vi "Periodic Tasks.vi"(8 "error in":errorcluster) -> ()   [LabVIEW 2017]
doc: "This VI runs in parallel to other tasks. It can contain as many user-defined periodic loops as you need. These can carry out PID or other sorts of timed response."
uses:
  <vilib>/Rock Robotics/WPI/Solenoid/WPI_SolenoidValue.ctl
  <vilib>/Rock Robotics/WPI/DriverStation/WPI_DriverStationRobotMode2.ctl
  <vilib>/Rock Robotics/WPI/ThirdParty/Phoenix-LabVIEW/Motor Controller/Controls/CTRE_Phoenix_MotorControl_ControlMode.ctl
  LabVIEW_is_Under_Control.lib/Util/Toggle/Change Detect.vi
  LabVIEW_is_Under_Control.lib/Util/Toggle/Change Detect Boolean.vi
  Robot Global Data.vi
  <vilib>/Rock Robotics/Network Tables/NT Write String.vi
  <vilib>/Rock Robotics/Network Tables/NT Write Number.vi
  <vilib>/Rock Robotics/WPI/Solenoid/WPI_SolenoidSetEnum.vi
  <vilib>/Rock Robotics/Network Tables/NT Write Boolean.vi
  <vilib>/Rock Robotics/Network Tables/NT Read Boolean.vi
panel:
  in  "Holding? Time":dbl=1000.0 format="%#_13g"
  out "Elevador Encoder":dbl
  out "Yaw":dbl
  in  "Exchange":dbl=4.0
  in  "ScoringHigh":dbl=80.0
  in  "Scoring Low":dbl=67.0
  in  "Enable squared":bool
  in  "Score":dbl=-0.3
  in  "Segurando":dbl=0.3
  in  "Expelir":dbl=-0.3
  in  "Coletar":dbl=0.9
  # "Para alterar:\n\nAlternar velocidade entre exchange e switch/scale\n\nNão deixar cancelar enquanto está cancelando"
  # "Intake"
  # "Drivetrain"
  # "Elevador"
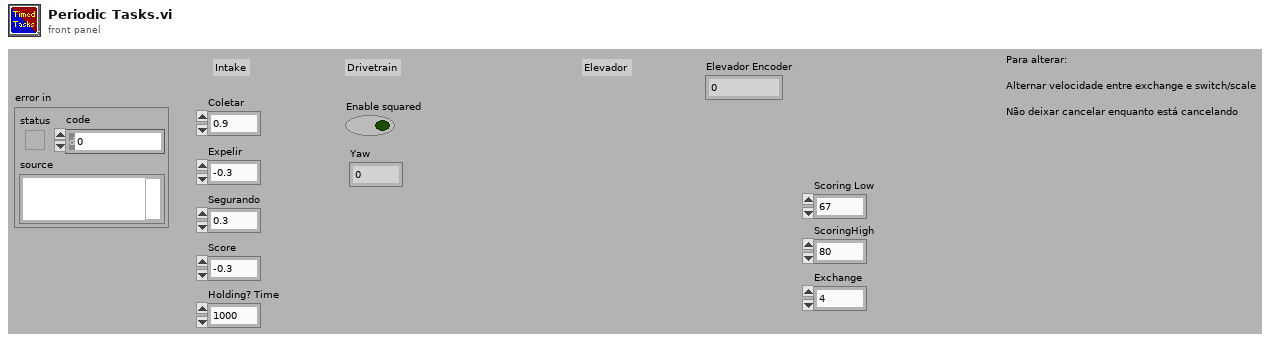
[diagram p1: front panel]
types:
  T1 = typedef "Máquina de estado do elevador.ctl" = enum16{"Resting", "Scoring Low", "Scoring Higher", "Exchange"}
  T2 = enum16{"Repouso", "Coletando", "Segurando", "Score"}
  T3 = typedef "WPI_EncoderDevRef.ctl" = cluster{"DevStatus":errorcluster, "EncoderIndex":T4, "CounterIndex":T5, "DistancePerCount":dbl, "Decoding Type":T6}
  T4 = typedef "FPGA_EncoderIdx.ctl" = enum8{"Enc 0", "Enc 1", "Enc 2", "Enc 3", "Enc 4", "Enc 5", "Enc 6", "Enc 7", "Invalid"}
  T5 = typedef "FPGA_CounterCtrSystemIndex.ctl" = enum8{"Ctr 0", "Ctr 1", "Ctr 2", "Ctr 3", "Ctr 4", "Ctr 5", "Ctr 6", "Ctr 7", "Invalid"}
  T6 = typedef "WPI_EncoderType.ctl" = enum16{"1x", "2x", "4x"}
  T7 = typedef "WPI_SwitchDevRef.ctl" = cluster{"DevStatus":errorcluster, "DIO Channel":T8, "CntIndex":T5, "Normally Closed":bool}
  T8 = typedef "FPGA_DIOChannel.ctl" = enum8{"DIO 0", "DIO 1", "DIO 2", "DIO 3", "DIO 4", "DIO 5", "DIO 6", "DIO 7", "DIO 8", "DIO 9", "DIO MXP 0", "DIO MXP 1", "DIO MXP 2", "DIO MXP 3", "DIO MXP 4", "DIO MXP 5", "DIO MXP 6", "DIO MXP 7", "DIO MXP 8", "DIO MXP 9", "DIO MXP 10", "DIO MXP 11", "DIO MXP 12", "DIO MXP 13", "DIO MXP 14", "DIO MXP 15", "SPI Port CS1", "SPI Port CS2", "SPI Port CS3", "SPI Port MISO", "SPI Port MOSI", "Invalid"}
  T9 = typedef "WPI_SolenoidDevRef.ctl" = cluster{"DevStatus":errorcluster, "Pneumatics Control Module":u8, "Forward Solenoid Channel":T10, "Reverse Solenoid Channel":T10}
  T10 = typedef "WPI_SolenoidChannel.ctl" = enum8{"Solenoid 0", "Solenoid 1", "Solenoid 2", "Solenoid 3", "Solenoid 4", "Solenoid 5", "Solenoid 6", "Solenoid 7", "Invalid"}
  T11 = typedef "WPI_MotorControlDeviceRef.ctl" = cluster{"DeviceStatus":errorcluster, "Type":T12, "PWM":cluster{"PWM Channel":T13, "DeadBand":T14}, "CAN":cluster{"Device Number":u8, "SetOutput VI Ref":variant, "GetOutput VI Ref":variant, "Enable VI Ref":variant, "Disable VI Ref":variant, "Data":variant}, "Invert":bool, "DIO PWM":cluster{"PWM \"Enable\" Channel":T13, "DIOChannel":T8, "PWM Rate":dbl}}
  T12 = typedef "WPI_MotorControlType.ctl" = enum16{"PWM", "CAN", "DIO PWM"}
  T13 = typedef "FPGA_DIOPWMChannel.ctl" = enum8{"PWM 0", "PWM 1", "PWM 2", "PWM 3", "PWM 4", "PWM 5", "PWM 6", "PWM 7", "PWM 8", "PWM 9", "PWM MXP 0", "PWM MXP 1", "PWM MXP 2", "PWM MXP 3", "PWM MXP 4", "PWM MXP 5", "PWM MXP 6", "PWM MXP 7", "PWM MXP 8", "PWM MXP 9", "Invalid"}
  T14 = typedef "WPI_PWMDeadband.ctl" = cluster{"Name":string, "maxPositivePwm":i32, "minPositivePwm":i32, "centerPwm":i32, "maxNegativePwm":i32, "minNegativePwm":i32, "angularRange":u16}
  T15 = cluster{"Yaw":dbl, "Roll":dbl, "Pitch":dbl, "Heading":dbl, "Fused Heading":dbl}
  T16 = typedef "WPI_SolenoidValue.ctl" = enum16{"Off", "On", "Forward", "Reverse"}
  T17 = typedef "WPI_DriverStationRobotMode2.ctl" = enum16{"Autonomous Disabled", "Autonomous Enabled", "Teleop Disabled", "Teleop Enabled", "Disconnected", "Finish", "Test Disabled", "Test Enabled", "Emergency Stopped"}
  T18 = typedef "Button Cluster.ctl" = cluster{"Buttons[0]":bool, "Buttons[1]":bool, "Buttons[2]":bool, "Buttons[3]":bool, "Buttons[4]":bool, "Buttons[5]":bool, "Buttons[6]":bool, "Buttons[7]":bool, "Buttons[8]":bool, "Buttons[9]":bool}
  T19 = typedef "CTRE_Phoenix_MotorControl_ControlMode.ctl" = u16
  T20 = typedef "Axes Cluster.ctl" = cluster{"Axes[0]":dbl, "Axes[1]":dbl, "Axes[2]":dbl, "Axes[3]":dbl, "Axes[4]":dbl, "Axes[5]":dbl, "Axes[6]":dbl, "Axes[7]":dbl, "Axes[8]":dbl}
  T21 = typedef "D-Pad.ctl" = cluster{"Top":bool, "Bottom":bool, "None":bool, "Right":bool, "Left":bool}
  T22 = cluster{"proportional gain (Kc)":dbl, "integral time (Ti, min)":dbl, "derivative time (Td, min)":dbl}
  T23 = enum16{"Coletar", "Expelir", "Chao", "Down", "Up", "Resting"}
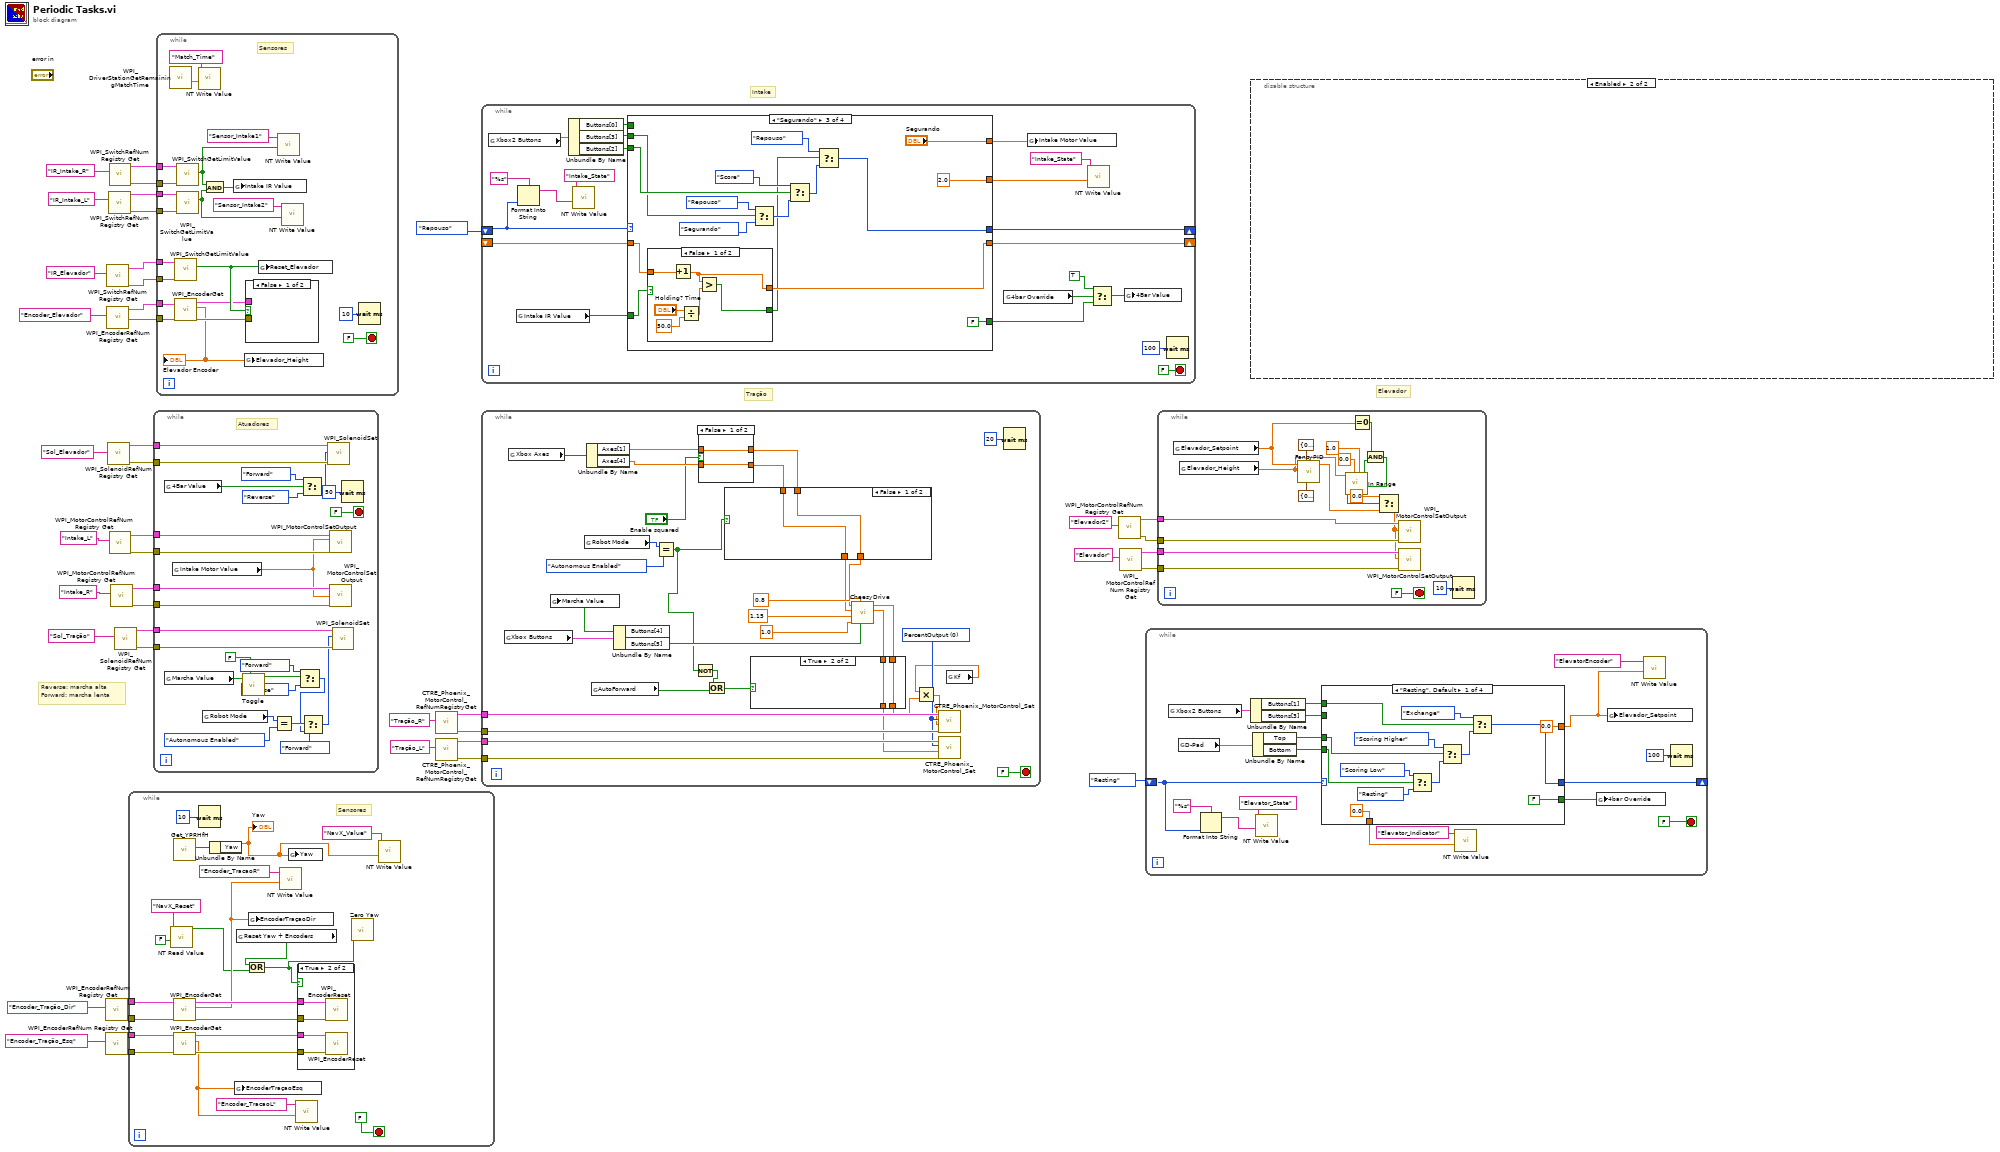
[diagram p0: block diagram]
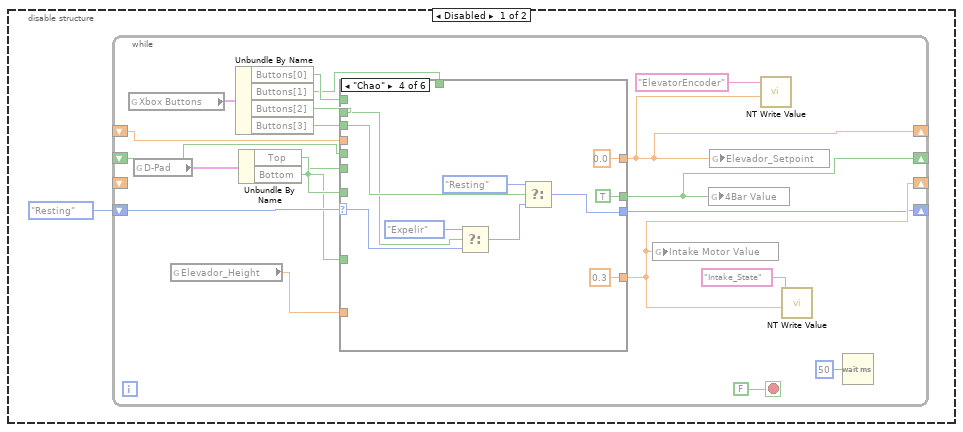
[diagram p2: hidden frame]
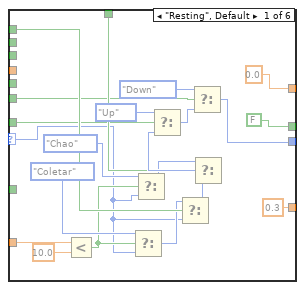
[diagram p3: hidden frame]
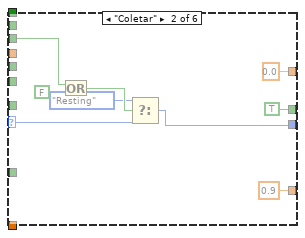
[diagram p4: hidden frame]
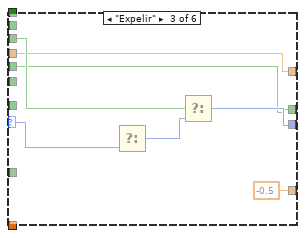
[diagram p5: hidden frame]
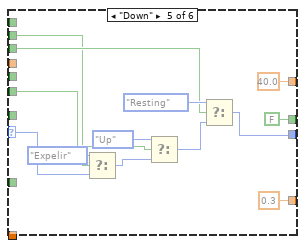
[diagram p6: hidden frame]
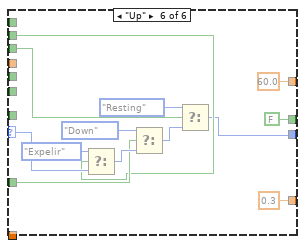
[diagram p7: hidden frame]
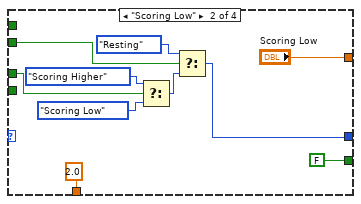
[diagram p9: hidden frame]
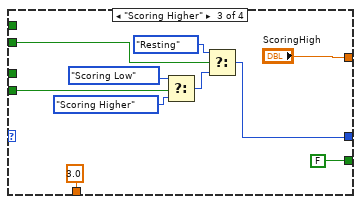
[diagram p10: hidden frame]
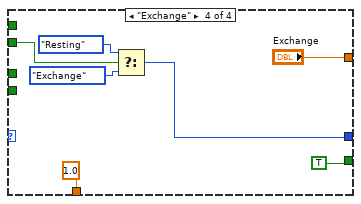
[diagram p11: hidden frame]
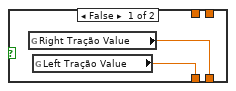
[diagram p12: hidden frame]
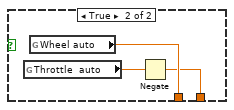
[diagram p13: hidden frame]
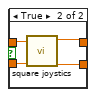
[diagram p14: hidden frame]
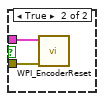
[diagram p15: hidden frame]
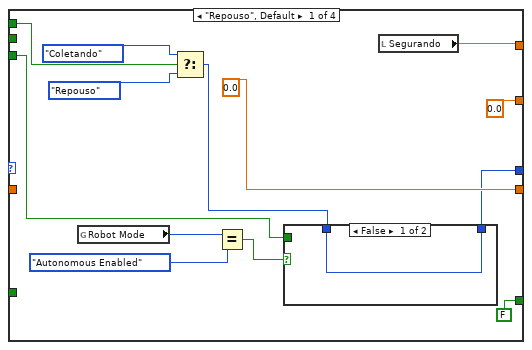
[diagram p16: hidden frame]
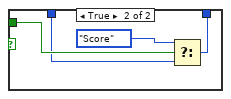
[diagram p17: hidden frame]
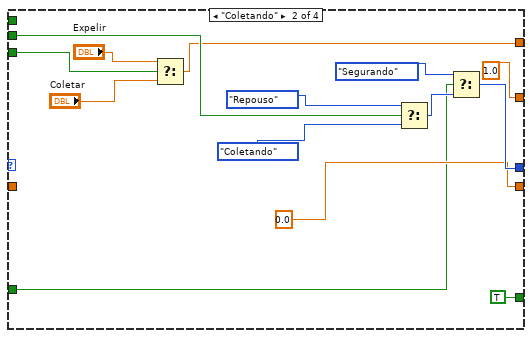
[diagram p18: hidden frame]
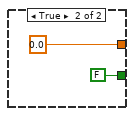
[diagram p19: hidden frame]
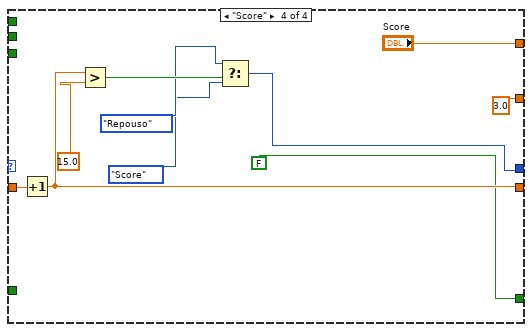
[diagram p20: hidden frame]
diagram:
  # "Reverse: marcha alta\nForward: marcha lenta"
  # "Elevador"
  # "Tração"
  # "Intake"
  n1 = call <vilib>:"WPI_EncoderRefNum Registry Get.vi"("refnum name"="Encoder_Tração_Dir") -> ("error out"=w8:errorcluster, "EncoderDevRef"=w9:T3)  [unwired: 9 in]
  n2 = call <vilib>:"WPI_EncoderRefNum Registry Get.vi"("refnum name"="Encoder_Tração_Esq") -> ("error out"=w7:errorcluster, "EncoderDevRef"=w6:T3)  [unwired: 9 in]
  n3 = call <vilib>:"WPI_SwitchRefNum Registry Get.vi"("refnum name"="IR_Elevador") -> ("error out"=w19:errorcluster, "SwitchDevRef"=w20:T7)  [unwired: 9 in]
  n4 = call <vilib>:"WPI_EncoderRefNum Registry Get.vi"("refnum name"="Encoder_Elevador") -> ("error out"=w15:errorcluster, "EncoderDevRef"=w16:T3)  [unwired: 9 in]
  n5 = call <vilib>:"WPI_SolenoidRefNum Registry Get.vi"("refnum name"="Sol_Elevador") -> ("error out"=w37:errorcluster, "SolenoidDevRef"=w36:T9)  [unwired: 9 in]
  n6 = call <vilib>:"WPI_SwitchRefNum Registry Get.vi"("refnum name"="IR_Intake_L") -> ("error out"=w42:errorcluster, "SwitchDevRef"=w41:T7)  [unwired: 9 in]
  n7 = call <vilib>:"WPI_SwitchRefNum Registry Get.vi"("refnum name"="IR_Intake_R") -> ("error out"=w40:errorcluster, "SwitchDevRef"=w39:T7)  [unwired: 9 in]
  n8 = call <vilib>:"WPI_MotorControlRefNum Registry Get.vi"("refnum name"="Intake_L") -> ("error out"=w35:errorcluster, "MotorControlDevRef"=w34:T11)  [unwired: 9 in]
  n9 = call <vilib>:"WPI_MotorControlRefNum Registry Get.vi"("refnum name"="Intake_R") -> ("error out"=w30:errorcluster, "MotorControlDevRef"=w31:T11)  [unwired: 9 in]
  n10 = call <vilib>:"WPI_SolenoidRefNum Registry Get.vi"("refnum name"="Sol_Tração") -> ("error out"=w27:errorcluster, "SolenoidDevRef"=w28:T9)  [unwired: 9 in]
  n11 = while {
    tunnel: w9 -> [w66]
    tunnel: w8 -> [w65]
    tunnel: w6 -> [w63]
    tunnel: w7 -> [w64]
    stop <- FALSE stop-if-true
    # "Sensores"
    n12 = call-poly <vilib>:"NT Read Value.vi"("Default Value"=FALSE, "Name"="NavX_Reset") -> ("Boolean"=w47:bool)  [unwired: 8 in, 1 out]
    n13 = call <vilib>:"Get_YPRHfH.vi"() -> ("YRPHfH"=w56:T15)  [unwired: 11 in]
    n14 = call <vilib>:"WPI_EncoderGet.vi"("error in (no error)"=w65, "EncoderDevRef"=w66) -> ("error out"=w59:errorcluster, "Distance"=w52:dbl, "EncoderDevRef"=w60:T3)  [unwired: 4 in, 3 out]
    n15 = call <vilib>:"WPI_EncoderGet.vi"("error in (no error)"=w64, "EncoderDevRef"=w63) -> ("error out"=w57:errorcluster, "Distance"=w54:dbl, "EncoderDevRef"=w58:T3)  [unwired: 4 in, 3 out]
    n16 = Wait (ms)(milliseconds to wait=u32 10) -> ()  [unwired: 1 out]
    n17 = Unbundle By Name(w56) -> ("Yaw"=w51:dbl)
    "Yaw" <- w51
    n18 = global write "Robot Global Data.vi" "EncoderTraçaoEsq"(w54) -> ()
    n19 = global read "Robot Global Data.vi" "Reset Yaw + Encoders"() -> (w48:bool)
    n20 = Or(x=w48, y=w47) -> (x .or. y?=w46:bool)
    n21 = global write "Robot Global Data.vi" "EncoderTraçaoDir"(w52) -> ()
    n22 = call-poly <vilib>:"NT Write Value.vi"("Numeric"=w52, "Name"="Encoder_TracaoR") -> ()  [unwired: 9 in, 1 out]
    n23 = global write "Robot Global Data.vi" "Yaw"(w51) -> ()
    n24 = call-poly <vilib>:"NT Write Value.vi"("Numeric"=w54, "Name"="Encoder_TracaoL") -> ()  [unwired: 9 in, 1 out]
    n25 = case shown="True" w46 {
      tunnel: w60 -> [_ w70]
      tunnel: w59 -> [_ w69]
      tunnel: w58 -> [_ w68]
      tunnel: w57 -> [_ w67]
      frame False {
      }
      frame True {
        n26 = call <vilib>:"WPI_EncoderReset.vi"("error in (no error)"=w69, "EncoderDevRef"=w70) -> ()  [unwired: 8 in, 2 out]
        n27 = call <vilib>:"WPI_EncoderReset.vi"("error in (no error)"=w67, "EncoderDevRef"=w68) -> ()  [unwired: 8 in, 2 out]
      }
    }
    n28 = call <vilib>:"Zero Yaw.vi"("Zero"=w46) -> ()  [unwired: 11 in]
    n29 = call-poly <vilib>:"NT Write Value.vi"("Numeric"=w51, "Name"="NavX_Value") -> ()  [unwired: 9 in, 1 out]
  }
  n30 = while {
    tunnel: w37 -> [w96]
    tunnel: w36 -> [w95]
    tunnel: w35 -> [w90]
    tunnel: w34 -> [w89]
    tunnel: w31 -> [w88]
    tunnel: w30 -> [w87]
    tunnel: w28 -> [w81]
    tunnel: w27 -> [w80]
    stop <- FALSE stop-if-true
    # "Atuadores"
    n31 = global read "Robot Global Data.vi" "4Bar Value"() -> (w91:bool)
    n32 = global read "Robot Global Data.vi" "Marcha Value"() -> (w79:bool)
    n33 = global read "Robot Global Data.vi" "Intake Motor Value"() -> (w86:dbl)
    n34 = global read "Robot Global Data.vi" "Robot Mode"() -> (w77:T17)
    n35 = call "Toggle.vi"("Initial Value"=FALSE, "In"=w79) -> ("Toggled"=w78:bool)  [unwired: 9 in]
    n36 = Equal?(x=w77, y=WPI_DriverStationRobotMode2."Autonomous Enabled") -> (x = y?=w75:bool)
    n37 = Select(t=WPI_SolenoidValue."Forward" ("Value"), s=w78, f=WPI_SolenoidValue."Reverse" ("Value")) -> (s? t:f=w72:T16)
    n38 = Select(t=WPI_SolenoidValue."Forward" ("Value"), s=w91, f=WPI_SolenoidValue."Reverse" ("Value")) -> (s? t:f=w94:T16)
    n39 = Select(t=WPI_SolenoidValue."Forward", s=w75, f=w72) -> (s? t:f=w73:T16)
    n40 = call-poly <vilib>:"WPI_SolenoidSet.vi"("error in (no error)"=w96, "Value"=w94, "SolenoidDevRef"=w95) -> ()  [unwired: 7 in, 2 out]
    n41 = call <vilib>:"WPI_MotorControlSetOutput.vi"("error in (no error)"=w87, "Output"=w86, "MotorControlDevRef"=w88) -> ()  [unwired: 6 in, 3 out]
    n42 = call <vilib>:"WPI_MotorControlSetOutput.vi"("error in (no error)"=w90, "Output"=w86, "MotorControlDevRef"=w89) -> ()  [unwired: 6 in, 3 out]
    n43 = call-poly <vilib>:"WPI_SolenoidSet.vi"("error in (no error)"=w80, "Value"=w73, "SolenoidDevRef"=w81) -> ()  [unwired: 7 in, 2 out]
    n44 = Wait (ms)(milliseconds to wait=u32 50) -> ()  [unwired: 1 out]
  }
  n45 = while {
    tunnel: w42 -> [w114]
    tunnel: w41 -> [w113]
    tunnel: w40 -> [w112]
    tunnel: w39 -> [w111]
    tunnel: w19 -> [w109]
    tunnel: w20 -> [w110]
    tunnel: w16 -> [w108]
    tunnel: w15 -> [w107]
    stop <- FALSE stop-if-true
    # "Sensores"
    n46 = call <vilib>:"WPI_DriverStationGetRemainingMatchTime.vi"() -> ("Match Time(s)"=w98:sgl)  [unwired: 10 in, 1 out]
    n47 = call <vilib>:"WPI_SwitchGetLimitValue.vi"("error in (no error)"=w109, "SwitchDevRef"=w110) -> ("Switch Pressed"=w106:bool)  [unwired: 7 in, 2 out]
    n48 = call <vilib>:"WPI_EncoderGet.vi"("error in (no error)"=w107, "EncoderDevRef"=w108) -> ("error out"=w104:errorcluster, "Distance"=w103:dbl, "EncoderDevRef"=w105:T3)  [unwired: 4 in, 3 out]
    "Elevador Encoder" <- w103
    n49 = call <vilib>:"WPI_SwitchGetLimitValue.vi"("error in (no error)"=w114, "SwitchDevRef"=w113) -> ("Switch Pressed"=w102:bool)  [unwired: 7 in, 2 out]
    n50 = call <vilib>:"WPI_SwitchGetLimitValue.vi"("error in (no error)"=w112, "SwitchDevRef"=w111) -> ("Switch Pressed"=w99:bool)  [unwired: 7 in, 2 out]
    n51 = call-poly <vilib>:"NT Write Value.vi"("Numeric"=w98, "Name"="Match_Time") -> ()  [unwired: 9 in, 1 out]
    n52 = And(x=w99, y=w102) -> (x .and. y?=w115:bool)
    n53 = global write "Robot Global Data.vi" "Intake IR Value"(w115) -> ()
    n54 = global write "Robot Global Data.vi" "Elevador_Height"(w103) -> ()
    n55 = case shown="False" w106 {
      tunnel: w105 -> [_ w119]
      tunnel: w104 -> [_ w118]
      frame False {
      }
      frame True {
        n56 = call <vilib>:"WPI_EncoderReset.vi"("error in (no error)"=w118, "EncoderDevRef"=w119) -> ()  [unwired: 8 in, 2 out]
      }
    }
    n57 = global write "Robot Global Data.vi" "Reset_Elevador"(w106) -> ()
    n58 = call-poly <vilib>:"NT Write Value.vi"("Boolean"=w99, "Name"="Sensor_Intake1") -> ()  [unwired: 9 in, 1 out]
    n59 = call-poly <vilib>:"NT Write Value.vi"("Boolean"=w102, "Name"="Sensor_Intake2") -> ()  [unwired: 9 in, 1 out]
    n60 = Wait (ms)(milliseconds to wait=u32 10) -> ()  [unwired: 1 out]
  }
  n61 = call <vilib>:"CTRE_Phoenix_MotorControl_RefNumRegistryGet.vi"("refnum name"="Tração_R") -> ("error out"=w22:errorcluster, "PhoenixMotorControlDevRef"=w24:T11)  [unwired: 9 in]
  n62 = call <vilib>:"CTRE_Phoenix_MotorControl_RefNumRegistryGet.vi"("refnum name"="Tração_L") -> ("error out"=w21:errorcluster, "PhoenixMotorControlDevRef"=w23:T11)  [unwired: 9 in]
  n63 = while {
    shift-right: [w137] -> _
    shift-left: T2."Repouso" -> [w123]
    shift-right: [w135] -> _
    shift-left: _ -> [w136]
    stop <- FALSE stop-if-true
    n64 = global read "Robot Global Data.vi" "Xbox2 Buttons"() -> (w138:T18)
    n65 = global read "Robot Global Data.vi" "Intake IR Value"() -> (w120:bool)
    n66 = Format Into String(format string="%s", w123) -> (resulting string=w122:string)  [unwired: 2 in, 1 out]
    n67 = Unbundle By Name(w138) -> ("Buttons[0]"=w131:bool, "Buttons[3]"=w133:bool, "Buttons[2]"=w132:bool)
    n68 = call-poly <vilib>:"NT Write Value.vi"("String"=w122, "Name"="Intake_State") -> ()  [unwired: 9 in, 1 out]
    n69 = case shown="\"Segurando\"" w123 {
      tunnel: w131 -> [w153 _ _ _]
      tunnel: [w144 w169 w173 w200] -> w137
      tunnel: w133 -> [_ w172 w187 _]
      tunnel: w132 -> [w143 w163 w188 _]
      tunnel: w136 -> [_ _ w177 w206]
      tunnel: [0.0 0.0 w178 w205] -> w135
      tunnel: [w141 w164 "Segurando" "Score"] -> w134
      tunnel: [FALSE TRUE FALSE FALSE] -> w125
      tunnel: [0.0 1.0 2.0 3.0] -> w127
      tunnel: w120 -> [_ w160 w179 _]
      frame "Repouso", Default {
        n70 = global read "Robot Global Data.vi" "Robot Mode"() -> (w147:T17)
        n71 = Select(t=T2."Coletando", s=w153, f=T2."Repouso") -> (s? t:f=w145:T2)
        n72 = Equal?(x=w147, y=WPI_DriverStationRobotMode2."Autonomous Enabled") -> (x = y?=w146:bool)
        n73 = case shown="False" w146 {
          tunnel: w143 -> [_ w158]
          tunnel: w145 -> [w154 w157]
          tunnel: [w154 w155] -> w144
          frame False {
          }
          frame True {
            n74 = Select(t=T2."Score", s=w158, f=w157) -> (s? t:f=w155:T2)
          }
        }
        n75 = local read "Segurando"() -> (w141:dbl)
      }
      frame "Coletando" {
        n76 = Select(t="Expelir", s=w163, f="Coletar") -> (s? t:f=w164:dbl)
        n77 = Select(t=T2."Repouso", s=w172, f=T2."Coletando") -> (s? t:f=w166:T2)
        n78 = Select(t=T2."Segurando", s=w160, f=w166) -> (s? t:f=w169:T2)
      }
      frame "Segurando" {
        n79 = case shown="False" w179 {
          tunnel: [w193 0.0] -> w178
          tunnel: w177 -> [w194 _]
          tunnel: [w192 FALSE] -> w174
          frame False {
            n80 = Increment(x=w194) -> (x+1=w193:dbl)
            n81 = Divide(x="Holding? Time", y=50.0) -> (x/y=w189:dbl)
            n82 = Greater?(x=w193, y=w189) -> (0:w192:bool)
          }
          frame True {
          }
        }
        n83 = Select(t=T2."Repouso", s=w187, f=T2."Segurando") -> (s? t:f=w186:T2)
        n84 = Select(t=T2."Score", s=w188, f=w186) -> (s? t:f=w176:T2)
        n85 = Select(t=T2."Repouso", s=w174, f=w176) -> (s? t:f=w173:T2)
      }
      frame "Score" {
        n86 = Increment(x=w206) -> (x+1=w205:dbl)
        n87 = Greater?(x=w205, y=15.0) -> (0:w203:bool)
        n88 = Select(t=T2."Repouso", s=w203, f=T2."Score") -> (s? t:f=w200:T2)
      }
    }
    n89 = global read "Robot Global Data.vi" "4bar Override"() -> (w130:bool)
    n90 = global write "Robot Global Data.vi" "Intake Motor Value"(w134) -> ()
    n91 = call-poly <vilib>:"NT Write Value.vi"("Numeric"=w127, "Name"="Intake_State") -> ()  [unwired: 9 in, 1 out]
    n92 = Select(t=TRUE, s=w130, f=w125) -> (s? t:f=w129:bool)
    n93 = global write "Robot Global Data.vi" "4Bar Value"(w129) -> ()
    n94 = Wait (ms)(milliseconds to wait=u32 100) -> ()  [unwired: 1 out]
  }
  n95 = while {
    tunnel: w24 -> [w230]
    tunnel: w23 -> [w229]
    tunnel: w22 -> [w228]
    tunnel: w21 -> [w227]
    stop <- FALSE stop-if-true
    w226 = T19 0 items=["PercentOutput"=0, "Position"=1, "Velocity"=2, "Current"=3, "Follower"=5, "MotionProfile"=6, "MotionMagic"=7, "MotionMagicArc"=8, "MotionProfileArc"=10, "Disabled"=15] ("Control Mode")
    n96 = global read "Robot Global Data.vi" "Xbox Buttons"() -> (w237:T18)
    n97 = global read "Robot Global Data.vi" "Xbox Axes"() -> (w239:T20)
    n98 = global read "Robot Global Data.vi" "Robot Mode"() -> (w222:T17)
    n99 = Unbundle By Name(w239) -> ("Axes[1]"=w224:dbl, "Axes[4]"=w225:dbl)
    n100 = global read "Robot Global Data.vi" "AutoForward"() -> (w211:bool)
    n101 = Unbundle By Name(w237) -> ("Buttons[4]"=w235:bool, "Buttons[5]"=w236:bool)
    n102 = global write "Robot Global Data.vi" "Marcha Value"(w235) -> ()
    n103 = Equal?(x=w222, y=WPI_DriverStationRobotMode2."Autonomous Enabled") -> (x = y?=w210:bool)
    n104 = Not(x=w210) -> (.not. x?=w213:bool)
    n105 = case shown="False" "Enable squared" {
      tunnel: w225 -> [w250 w254]
      tunnel: [w250 w253] -> w219
      tunnel: w224 -> [w249 w252]
      tunnel: [w249 w251] -> w220
      frame False {
      }
      frame True {
        n106 = call "square joystics.vi"("right joy"=w254, "left joy"=w252) -> ("Right Out"=w253:dbl, "Left Out"=w251:dbl)  [unwired: 8 in]
      }
    }
    n107 = Or(x=w213, y=w211) -> (x .or. y?=w212:bool)
    n108 = case shown="False" w210 {
      tunnel: [w244 w248] -> w214
      tunnel: [w245 w246] -> w215
      tunnel: w220 -> [w245 _]
      tunnel: w219 -> [w244 _]
      frame False {
      }
      frame True {
        n109 = global read "Robot Global Data.vi" "Throttle  auto"() -> (w247:dbl)
        n110 = global read "Robot Global Data.vi" "Wheel auto"() -> (w248:dbl)
        n111 = Negate(x=w247) -> (-x=w246:dbl)
      }
    }
    n112 = call "CheesyDrive.vi"("Quickturn"=w236, "WheelNonLinearity"=0.8, "negInertiaScalar"=1.0, "Sensitivty"=1.15, "Wheel"=w214, "Throttle"=w215) -> ("Right PWM"=w216:dbl, "Left PWM"=w218:dbl)  [unwired: 4 in]
    n113 = case shown="True" w212 {
      tunnel: [w240 w242] -> w209
      tunnel: w218 -> [_ w242]
      tunnel: [w241 w243] -> w217
      tunnel: w216 -> [_ w243]
      frame False {
        n114 = global read "Robot Global Data.vi" "Right Tração Value"() -> (w240:dbl)
        n115 = global read "Robot Global Data.vi" "Left Tração Value"() -> (w241:dbl)
      }
      frame True {
      }
    }
    n116 = call <vilib>:"CTRE_Phoenix_MotorControl_Set.vi"("error in (no error)"=w227, "Output"=w217, "Control Mode"=w226, "PhoenixMotorControlDevRef"=w229) -> ()  [unwired: 6 in, 2 out]
    n117 = global read "Robot Global Data.vi" "Kf"() -> (w208:dbl)
    n118 = Multiply(x=w208, y=w209) -> (x*y=w207:dbl)
    n119 = call <vilib>:"CTRE_Phoenix_MotorControl_Set.vi"("error in (no error)"=w228, "Output"=w207, "Control Mode"=w226, "PhoenixMotorControlDevRef"=w230) -> ()  [unwired: 6 in, 2 out]
    n120 = Wait (ms)(milliseconds to wait=u32 20) -> ()  [unwired: 1 out]
  }
  n121 = call <vilib>:"WPI_MotorControlRefNum Registry Get.vi"("refnum name"="Elevador2") -> ("error out"=w2:errorcluster, "MotorControlDevRef"=w3:T11)  [unwired: 9 in]
  n122 = call <vilib>:"WPI_MotorControlRefNum Registry Get.vi"("refnum name"="Elevador") -> ("error out"=w12:errorcluster, "MotorControlDevRef"=w13:T11)  [unwired: 9 in]
  n123 = while {
    shift-right: [w270] -> _
    shift-left: Máquina_de_estado_do_elevador."Resting" -> [w255]
    stop <- FALSE stop-if-true
    n124 = global read "Robot Global Data.vi" "Xbox2 Buttons"() -> (w264:T18)
    n125 = global read "Robot Global Data.vi" "D-Pad"() -> (w263:T21)
    n126 = Format Into String(format string="%s", w255) -> (resulting string=w257:string)  [unwired: 2 in, 1 out]
    n127 = Unbundle By Name(w264) -> ("Buttons[1]"=w262:bool, "Buttons[3]"=w261:bool)
    n128 = Unbundle By Name(w263) -> ("Top"=w260:bool, "Bottom"=w259:bool)
    n129 = call-poly <vilib>:"NT Write Value.vi"("String"=w257, "Name"="Elevator_State") -> ()  [unwired: 9 in, 1 out]
    n130 = case shown="\"Resting\", Default" w255 {
      tunnel: [0.0 ("Exchange") "Scoring Low" "ScoringHigh" "Exchange"] -> w265
      tunnel: [w279 w293 w303 w311] -> w270
      tunnel: [FALSE FALSE FALSE TRUE] -> w269
      tunnel: [0.0 2.0 3.0 1.0] -> w267
      tunnel: w262 -> [w276 _ _ _]
      tunnel: w261 -> [_ w286 w296 w306]
      tunnel: w260 -> [w275 w287 _ _]
      tunnel: w259 -> [w274 _ w297 _]
      frame "Resting", Default {
        n131 = Select(t=Máquina_de_estado_do_elevador."Scoring Low", s=w274, f=Máquina_de_estado_do_elevador."Resting") -> (s? t:f=w285:T1)
        n132 = Select(t=Máquina_de_estado_do_elevador."Scoring Higher", s=w275, f=w285) -> (s? t:f=w284:T1)
        n133 = Select(t=Máquina_de_estado_do_elevador."Exchange", s=w276, f=w284) -> (s? t:f=w279:T1)
      }
      frame "Scoring Low" {
        n134 = Select(t=Máquina_de_estado_do_elevador."Scoring Higher", s=w287, f=Máquina_de_estado_do_elevador."Scoring Low") -> (s? t:f=w294:T1)
        n135 = Select(t=Máquina_de_estado_do_elevador."Resting", s=w286, f=w294) -> (s? t:f=w293:T1)
      }
      frame "Scoring Higher" {
        n136 = Select(t=Máquina_de_estado_do_elevador."Scoring Low", s=w297, f=Máquina_de_estado_do_elevador."Scoring Higher") -> (s? t:f=w304:T1)
        n137 = Select(t=Máquina_de_estado_do_elevador."Resting", s=w296, f=w304) -> (s? t:f=w303:T1)
      }
      frame "Exchange" {
        n138 = Select(t=Máquina_de_estado_do_elevador."Resting", s=w306, f=Máquina_de_estado_do_elevador."Exchange") -> (s? t:f=w311:T1)
      }
    }
    n139 = call-poly <vilib>:"NT Write Value.vi"("Numeric"=w267, "Name"="Elevator_Indicator") -> ()  [unwired: 9 in, 1 out]
    n140 = global write "Robot Global Data.vi" "4bar Override"(w269) -> ()
    n141 = global write "Robot Global Data.vi" "Elevador_Setpoint"(w265) -> ()
    n142 = call-poly <vilib>:"NT Write Value.vi"("Numeric"=w265, "Name"="ElevatorEncoder") -> ()  [unwired: 9 in, 1 out]
    n143 = Wait (ms)(milliseconds to wait=u32 100) -> ()  [unwired: 1 out]
  }
  n144 = while {
    tunnel: w13 -> [w328]
    tunnel: w12 -> [w327]
    tunnel: w3 -> [w324]
    tunnel: w2 -> [w323]
    stop <- FALSE stop-if-true
    n145 = global read "Robot Global Data.vi" "Elevador_Setpoint"() -> (w322:dbl)
    n146 = global read "Robot Global Data.vi" "Elevador_Height"() -> (w315:dbl)
    n147 = call "FancyPID.vi"("Gains"=T22 {"proportional gain (Kc)"=0.095, "integral time (Ti, min)"=0.007, "derivative time (Td, min)"=0.0} ("Gains Elevador"), "Range"=cluster{"output high":dbl, "output low":dbl} {"output high"=0.95, "output low"=-0.25} ("Range Elevador"), "Process variable"=w315, "Setpoint"=w322) -> ("output"=w319:dbl)  [unwired: 7 in]
    n148 = call "In Range.vi"("Range"=1.0, "Setpoint"=0.0, "Value"=w315) -> ("in range?"=w316:bool)  [unwired: 8 in]
    n149 = Equal To 0?(x=w322) -> (x = 0?=w321:bool)
    n150 = And(x=w321, y=w316) -> (x .and. y?=w320:bool)
    n151 = Select(t=0.0, s=w320, f=w319) -> (s? t:f=w317:dbl)
    n152 = call <vilib>:"WPI_MotorControlSetOutput.vi"("error in (no error)"=w327, "Output"=w317, "MotorControlDevRef"=w328) -> ()  [unwired: 6 in, 3 out]
    n153 = call <vilib>:"WPI_MotorControlSetOutput.vi"("error in (no error)"=w323, "Output"=w317, "MotorControlDevRef"=w324) -> ()  [unwired: 6 in, 3 out]
    n154 = Wait (ms)(milliseconds to wait=u32 10) -> ()  [unwired: 1 out]
  }
  n155 = disable-structure shown="Enabled" {
    frame Disabled {
      n156 = while {
        shift-right: [w339] -> _
        shift-left: T23."Resting" -> [w350]
        shift-right: [w344] -> _
        shift-left: _ -> [w333]
        shift-right: [w343] -> _
        shift-left: _ -> [w332]
        shift-right: [w342] -> _
        shift-left: _ -> [_]
        stop <- FALSE stop-if-true
        n157 = global read "Robot Global Data.vi" "Xbox Buttons"() -> (w347:T18)
        n158 = global read "Robot Global Data.vi" "D-Pad"() -> (w346:T21)
        n159 = global read "Robot Global Data.vi" "Elevador_Height"() -> (w338:dbl)
        n160 = Unbundle By Name(w347) -> ("Buttons[0]"=w345:bool, "Buttons[1]"=w341:bool, "Buttons[2]"=w336:bool, "Buttons[3]"=w337:bool)
        n161 = Unbundle By Name(w346) -> ("Top"=w340:bool, "Bottom"=w335:bool)
        n162 = case shown="\"Chao\"" w350 {
          selector: w350 -> [w352 w375 w387 w392 w406 w420]
          tunnel: [0.0 0.0 w383 0.0 40.0 60.0] -> w344
          tunnel: [FALSE TRUE w382 TRUE FALSE FALSE] -> w343
          tunnel: [0.3 0.9 -0.5 0.3 0.3 0.3] -> w342
          tunnel: w345 -> [w367 _ _ _ _ _]
          tunnel: w341 -> [w365 _ _ _ _ _]
          tunnel: w340 -> [w364 _ _ _ _ _]
          tunnel: w335 -> [w362 _ _ _ w402 _]
          tunnel: [w360 w373 w385 w389 w407 w412] -> w339
          tunnel: w338 -> [w355 _ _ _ _ _]
          tunnel: w337 -> [_ w376 w388 w395 w403 w421]
          tunnel: w336 -> [_ _ _ w390 w400 w413]
          tunnel: w335 -> [_ _ _ _ _ w414]
          tunnel: w333 -> [_ _ w383 _ _ _]
          tunnel: w332 -> [_ _ w382 _ _ _]
          frame "Resting", Default {
            n163 = Less?(x=w355, y=10.0) -> (x < y?=w353:bool)
            n164 = Select(t=T23."Coletar", s=w353, f=w352) -> (s? t:f=w356:T23)
            n165 = Select(t=T23."Chao", s=w353, f=w352) -> (s? t:f=w358:T23)
            n166 = Select(t=w356, s=w367, f=w352) -> (s? t:f=w369:T23)
            n167 = Select(t=w358, s=w365, f=w369) -> (s? t:f=w368:T23)
            n168 = Select(t=T23."Up", s=w364, f=w368) -> (s? t:f=w366:T23)
            n169 = Select(t=T23."Down", s=w362, f=w366) -> (s? t:f=w360:T23)
          }
          frame "Coletar" {
            n170 = Or(x=w376, y=FALSE) -> (x .or. y?=w378:bool)
            n171 = Select(t=T23."Resting", s=w378, f=w375) -> (s? t:f=w373:T23)
          }
          frame "Expelir" {
            n172 = Select(f=w387) -> (s? t:f=w386:T23)  [unwired: 2 in]
            n173 = Select(s=w388, f=w386) -> (s? t:f=w385:T23)  [unwired: 1 in]
          }
          frame "Chao" {
            n174 = Select(t=T23."Expelir", s=w390, f=w392) -> (s? t:f=w393:T23)
            n175 = Select(t=T23."Resting", s=w395, f=w393) -> (s? t:f=w389:T23)
          }
          frame "Down" {
            n176 = Select(t=T23."Expelir", s=w400, f=w406) -> (s? t:f=w405:T23)
            n177 = Select(t=T23."Up", s=w402, f=w405) -> (s? t:f=w404:T23)
            n178 = Select(t=T23."Resting", s=w403, f=w404) -> (s? t:f=w407:T23)
          }
          frame "Up" {
            n179 = Select(t=T23."Expelir", s=w413, f=w420) -> (s? t:f=w419:T23)
            n180 = Select(t=T23."Down", s=w414, f=w419) -> (s? t:f=w418:T23)
            n181 = Select(t=T23."Resting", s=w421, f=w418) -> (s? t:f=w412:T23)
          }
        }
        n182 = global write "Robot Global Data.vi" "Intake Motor Value"(w342) -> ()
        n183 = global write "Robot Global Data.vi" "4Bar Value"(w343) -> ()
        n184 = global write "Robot Global Data.vi" "Elevador_Setpoint"(w344) -> ()
        n185 = call-poly <vilib>:"NT Write Value.vi"("Numeric"=w344, "Name"="ElevatorEncoder") -> ()  [unwired: 9 in, 1 out]
        n186 = call-poly <vilib>:"NT Write Value.vi"("Numeric"=w342, "Name"="Intake_State") -> ()  [unwired: 9 in, 1 out]
        n187 = Wait (ms)(milliseconds to wait=u32 50) -> ()  [unwired: 1 out]
      }
    }
    frame Enabled {
    }
  }
